vi "fgt set power.vi"(8 "error in (no error)":errorcluster, 10 "powerState":T1, 11 "controllerIndex":u16) -> (0 "error out":errorcluster)   [LabVIEW 2020, in "fgt_SDK.lvlib"]
doc: "Set power ON or OFF on a controller (such as Link, MFCS, Flowboard).\nNot all controllers support this functionality."
uses:
  fgt_SDK.lvlib
  TypeDefs/fgt_POWER.ctl
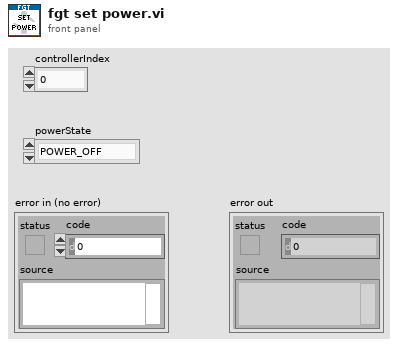
[diagram p1: front panel]
types:
  T1 = typedef "fgt_SDK.lvlib/fgt_POWER.ctl" = enum8{"POWER_OFF", "POWER_ON", "SLEEP"}
  T2 = typedef "fgt_SDK.lvlib/fgt_STATUS_INFO.ctl" = cluster{"InstrType":T3, "instrSN":u16, "errorCode":u8, "infoCode":u8, "detail":string}
  T3 = typedef "fgt_SDK.lvlib/fgt_INSTRUMENT_TYPE.ctl" = enum32{"None", "MFCS", "MFCS_EZ", "FRP", "LineUP", "IPS"}
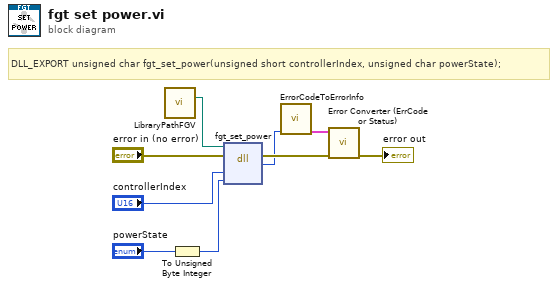
[diagram p0: block diagram]
diagram:
  # "DLL_EXPORT unsigned char fgt_set_power(unsigned short controllerIndex, unsigned char powerState);"
  n1 = call "LibraryPathFGV.vi"() -> ("Path Out"=w1:path)  [unwired: 14 in, 1 out]
  n2 = To Unsigned Byte Integer(number="powerState") -> (unsigned 8bit integer=w4:u8)
  n3 = dll-call lib="C:/Workspace/fgt-SDK/LabVIEW/dlls/fgt_SDK_*.*" fn="fgt_set_power"(path in=w1, error in="error in (no error)", "controllerIndex"="controllerIndex", "powerState"=w4) -> (error out=w7:errorcluster, "return type"=w3:u8)  [unwired: 3 in, 1 out]
  n4 = call "ErrorCodeToErrorInfo.vi"("return type"=w3) -> ("StatusInfo"=w2:T2)  [unwired: 10 in]
  n5 = call "Error Converter (ErrCode or Status).vi"("error in (no error)"=w7, "StatusInfo"=w2) -> ("error out"=→"error out":errorcluster)  [unwired: 9 in]
